vi "TDMS Logger.vi"() -> ()   [LabVIEW 2009]
panel:
  out "Données temporelles":waveform(dbl)[](graph)
  out "Spectre de puissance":waveform(dbl)[](graph)
  in  "Numéros de série UUT":string[](array[string])
  in  "Opérateur de test":string
  in  "Chemin du fichier TDMS":path=path "C:/Exercises/LabVIEW Core 2/TDMS Logger/Test Data.tdms"
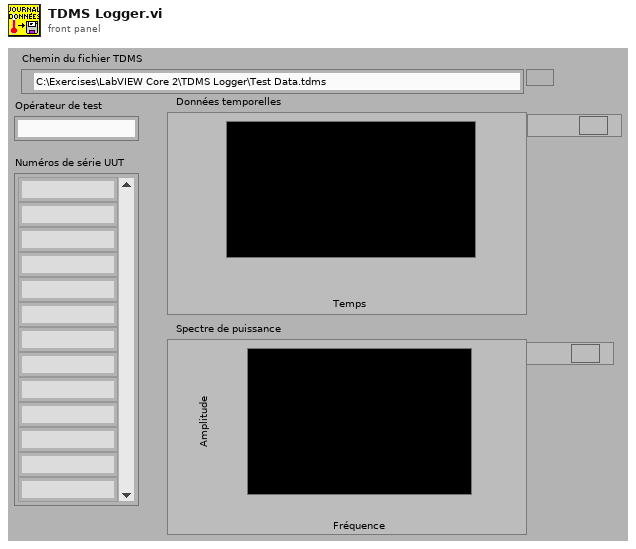
[diagram p1: front panel]
types:
  T1 = enum16{"open", "open or create", "create or replace", "create", "open (read-only)"}
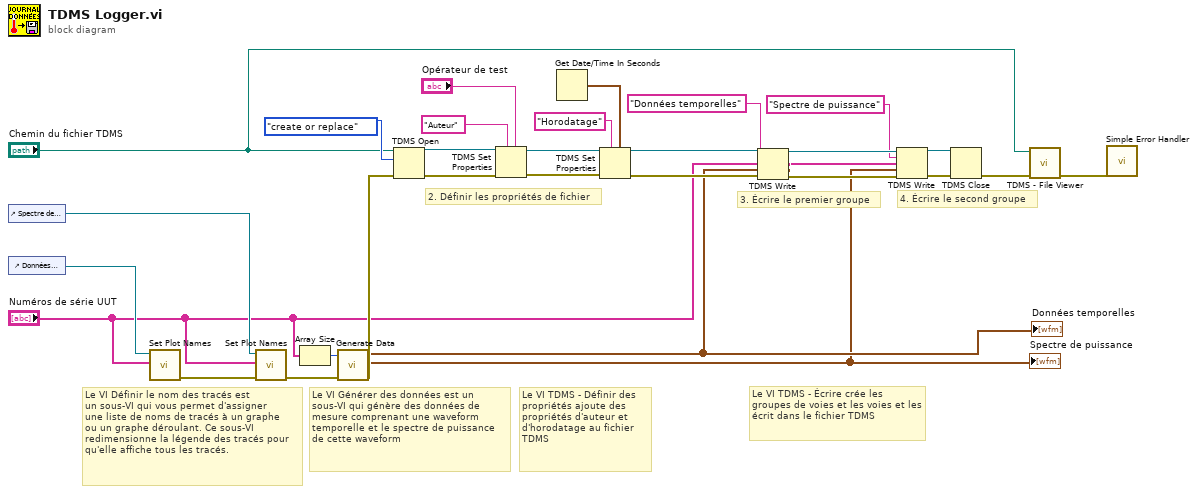
[diagram p0: block diagram]
diagram:
  # "4. Écrire le second groupe"
  # "3. Écrire le premier groupe"
  # "2. Définir les propriétés de fichier"
  # "Le VI TDMS - Définir des  propriétés ajoute des propriétés d'auteur et d'horodatage au fichier TDMS"
  # "Le VI TDMS - Écrire crée les groupes de voies et les voies et les écrit dans le fichier TDMS"
  # "Le VI Générer des données est un sous-VI qui génère des données de mesure comprenant une waveform temporelle et le spectre de puissance de cette waveform"
  # "Le VI Définir le nom des tracés est \nun sous-VI qui vous permet d'assigner \nune liste de noms de tracés à un graphe \nou un graphe déroulant. Ce sous-VI redimensionne la légende des tracés pour qu'elle affiche tous les tracés."
  n1 = control-ref of="Spectre de puissance"() -> (w30:refnum<vi>)
  n2 = control-ref of="Données temporelles"() -> (w26:refnum<vi>)
  n3 = call "Set Plot Names.vi"("Noms des tracés"="Numéros de série UUT", "Référence au graphe"=w26) -> ("sortie d'erreur"=w29:errorcluster)  [unwired: 9 in]
  n4 = call "Set Plot Names.vi"("entrée d'erreur (pas d'erreur)"=w29, "Noms des tracés"="Numéros de série UUT", "Référence au graphe"=w30) -> ("sortie d'erreur"=w27:errorcluster)  [unwired: 8 in]
  n5 = Array Size ("Taille d'un tableau")(array="Numéros de série UUT") -> (size(s)=w28:i32)
  n6 = call "Generate Data.vi"("entrée d'erreur"=w27, "Nombre de voies"=w28) -> ("sortie d'erreur"=w24:errorcluster, "Spectre de puissance"=w9:waveform(dbl)[], "Graphe déroulant"=w13:waveform(dbl)[])  [unwired: 7 in]
  "Spectre de puissance" <- w9
  "Données temporelles" <- w13
  n7 = TDMS Open ("TDMS - Ouvrir")(8:w24, 10:T1."create or replace" ("operation (0:open)"), 11:"Chemin du fichier TDMS") -> (0:w18:errorcluster, 3:w23:refnum<k34>)  [unwired: 3 in]
  n8 = TDMS Set Properties ("TDMS - Définir des propriétés")(5:"Opérateur de test", 7:"Auteur", 8:w18, 11:w23) -> (0:w22:errorcluster, 3:w21:refnum<k34>)  [unwired: 2 in, 2 out]
  n9 = Get Date/Time In Seconds ("Date et heure en secondes")() -> (seconds since 1Jan1904=w19:timestamp)
  n10 = TDMS Set Properties ("TDMS - Définir des propriétés")(5:w19, 7:"Horodatage" ("Title"), 8:w22, 11:w21) -> (0:w16:errorcluster, 3:w17:refnum<k34>)  [unwired: 2 in, 2 out]
  n11 = TDMS Write ("TDMS - Écrire")(0:w17, 5:"Données temporelles" ("group name in (Untitled)"), 7:"Numéros de série UUT", 9:w13, 11:w16) -> (4:w12:refnum<k34>, 8:w8:string[], 15:w11:errorcluster)  [unwired: 1 in, 1 out]
  n12 = TDMS Write ("TDMS - Écrire")(0:w12, 5:"Spectre de puissance" ("group name in (Untitled)"), 7:w8, 9:w9, 11:w11) -> (4:w7:refnum<k34>, 15:w6:errorcluster)  [unwired: 1 in, 2 out]
  n13 = TDMS Close ("TDMS - Fermer")(8:w6, 11:w7) -> (0:w5:errorcluster)
  n14 = call <vilib>:"TDMS - File Viewer.vi"("error in (no error)"=w5, "file path"="Chemin du fichier TDMS") -> ("error out"=w3:errorcluster)  [unwired: 4 in, 1 out]
  n15 = call <vilib>:"Simple Error Handler.vi"("error in (no error)"=w3) -> ()  [unwired: 4 in, 5 out]
